vi "Untitled 6.vi"   [LabVIEW 2013]
uses:
  <vilib>/NXT/Dual Mode Library/Waits/Wait_Num.vi
  <vilib>/NXT/Dual Mode Library/Advanced/NXTFlag_Assign.vi
types:
  T1 = typedef "LVHSConnector.ctl" = refnum<class "BrickReference.lvclass">
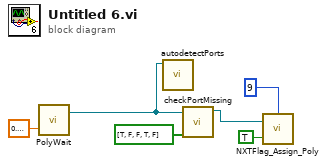
[diagram p0: block diagram]
diagram:
  n1 = call-poly <vilib>:"PolyWait.vi"("Time (1 sec)"=sgl 0.1) -> ("NXT/EV3"=w5:T1)  [unwired: 3 in]
  n2 = call "autodetectPorts.vi"("NXT/EV3"=w5) -> ()  [unwired: 11 in]
  n3 = call "checkPortMissing.vi"("Required"=bool[] [TRUE, FALSE, FALSE, TRUE, FALSE], "NXT/EV3"=w5) -> ("NXT/EV3"=w1:T1)  [unwired: 9 in]
  n4 = call-poly <vilib>:"NXTFlag_Assign_Poly.vi"("Flag State"=TRUE, "NXT/EV3"=w1, "NXT/EV3 Flag Number"=i8 9) -> ()  [unwired: 1 in, 1 out]
